vi "TestStand, RunState Fields, Scalar.vi"() -> (14 "Measurement Name":string, 15 "Low Limit":string, 16 "High Limit":string, 17 "Units":string, 18 "Comp":string)   [LabVIEW 2010]
doc: "Creates strings with TestStand Numeric Test Property Names."
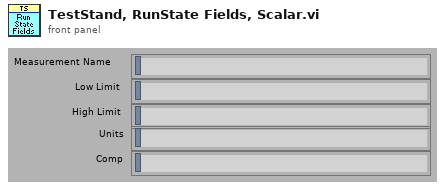
[diagram p1: front panel]
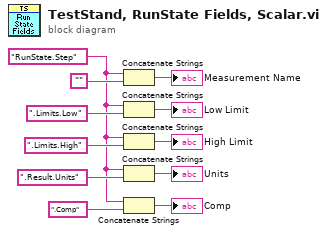
[diagram p0: block diagram]
diagram:
  w1 = "RunState.Step" ("suffix")
  n1 = Concatenate Strings(w1, "" ("prefix")) -> (→"Measurement Name":string)
  n2 = Concatenate Strings(w1, ".Limits.Low" ("prefix")) -> (→"Low Limit":string)
  n3 = Concatenate Strings(w1, ".Limits.High" ("prefix")) -> (→"High Limit":string)
  n4 = Concatenate Strings(w1, ".Result.Units" ("prefix")) -> (→"Units":string)
  n5 = Concatenate Strings(w1, ".Comp" ("prefix")) -> (→"Comp":string)
